vi "PeriodTasksNew.vi"() -> ()   [LabVIEW 2014]
panel:
  in  "Power Shaping Degree":dbl=2.0
  in  "Power Shaping Gain":dbl=50.0
  in  "Robot Width":dbl=27.25
  in  "Robot Length":dbl=19.875
  in  "Encoder Offset":dbl
  in  "EncoderTicksPerRev":dbl=1988.0
  in  "error in":errorcluster
  out "FL Angle":dbl=496.99998
  out "FR Angle":dbl=496.99998
  out "BL Angle":dbl=496.99998
  out "BR Angle":dbl=496.99998
  out "FL Power":dbl
  out "FR Power":dbl
  out "BL Power":dbl
  out "BR Power":dbl
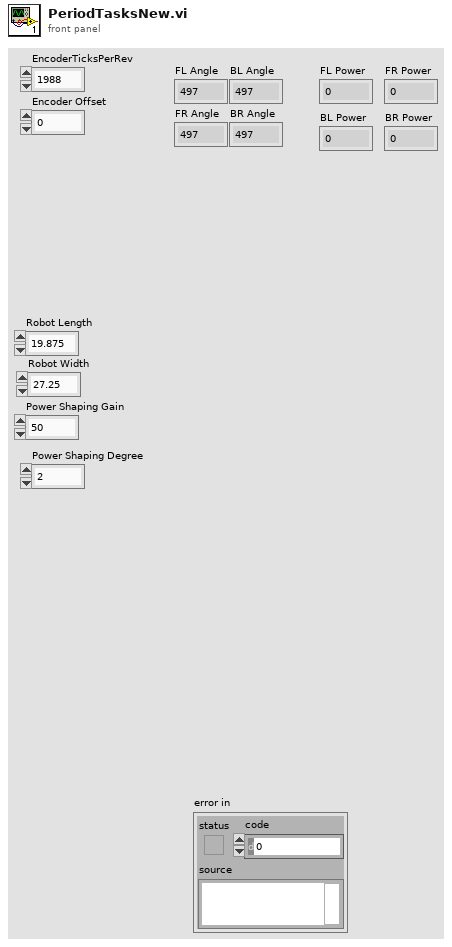
[diagram p1: front panel]
types:
  T1 = typedef "WPI_I2CDevRef.ctl" = cluster{"DevStatus":errorcluster, "Controller":T2, "Device Address":u8, "Handle":i32, "I2C Bus":T3}
  T2 = typedef "FPGA_TypedefDigitalModule.ctl" = enum16{"Controller 1"}
  T3 = typedef "i2c_bus.ctl" = enum16{"I2C On-Board", "I2C MXP", "Invalid"}
  T4 = typedef "WPI_MotorControlDeviceRef.ctl" = cluster{"DeviceStatus":errorcluster, "Type":T5, "PWM":cluster{"Controller":T2, "PWM Channel":T6, "DeadBand":T7}, "CAN":cluster{"Device Number":u8, "Control Mode":T8, "Semaphore":T9, "Max Vout":dbl, "TalonSRX Control Mode":T10}, "Invert":bool, "TransformRef":T11, "InvTransformRef":T11}
  T5 = typedef "WPI_MotorControlType.ctl" = enum16{"PWM", "CAN", "CANTalonSRX"}
  T6 = typedef "FPGA_DIOPWMChannel.ctl" = enum8{"PWM 0", "PWM 1", "PWM 2", "PWM 3", "PWM 4", "PWM 5", "PWM 6", "PWM 7", "PWM 8", "PWM 9", "PWM MXP 0", "PWM MXP 1", "PWM MXP 2", "PWM MXP 3", "PWM MXP 4", "PWM MXP 5", "PWM MXP 6", "PWM MXP 7", "PWM MXP 8", "PWM MXP 9", "Invalid"}
  T7 = typedef "WPI_PWMDeadband.ctl" = cluster{"Name":string, "maxPositivePwm":i32, "minPositivePwm":i32, "centerPwm":i32, "maxNegativePwm":i32, "minNegativePwm":i32, "angularRange":u16}
  T8 = typedef "WPI_CANJaguar_ControlMode.ctl" = enum8{"Percent VBus", "Current", "Speed", "Position", "Voltage"}
  T9 = typedef "Semaphore RefNum" = refnum<k1>
  T10 = typedef "WPI_CANTalonSRX_APIControlMode.ctl" = enum8{"Percent VBus", "Speed", "Position", "Slave", "Unchanged / Invalid"}
  T11 = typedef "WPI_PWMTransform_ConPane.ctl" = refnum<vi>
  T12 = typedef "WPI_JoystickDevRef.ctl" = cluster{"Device":T13}
  T13 = typedef "WPI_JoystickDeviceEnum.ctl" = enum16{"USB 0", "USB 1", "USB 2", "USB 3", "USB 4", "USB 5"}
  T14 = typedef "WPI_CANTalonSRX_GlobalStatus.ctl" = cluster{"Applied Throttle":dbl, "Module Enabled":bool, "CAN Error":errorcluster, "Closed Loop Error":dbl, "Forward Limit Switch Closed":bool, "Reverse Limit Switch Closed":bool, "Sensor Position":dbl, "Sensor Velocity":dbl, "Current":dbl, "Sticky Fault - Over Temp":bool, "Sticky Fault - Under Voltage":bool, "Sticky Fault - Forward Limit":bool, "Sticky Fault - Reverse Limit":bool, "Sticky Fault - Forward Soft Limit":bool, "Sticky Fault - Reverse Soft Limit":bool, "Brake is Enabled":bool, "Encoder Position":dbl, "Encoder Velocity":dbl, "Encoder Index Count":dbl, "Encoder A Pin State":bool, "Encoder B Pin State":bool, "Encoder Index Pin State":bool, "Analog In":dbl, "Analog In Velocity":dbl, "Temperature (C)":dbl, "Battery Voltage":dbl}
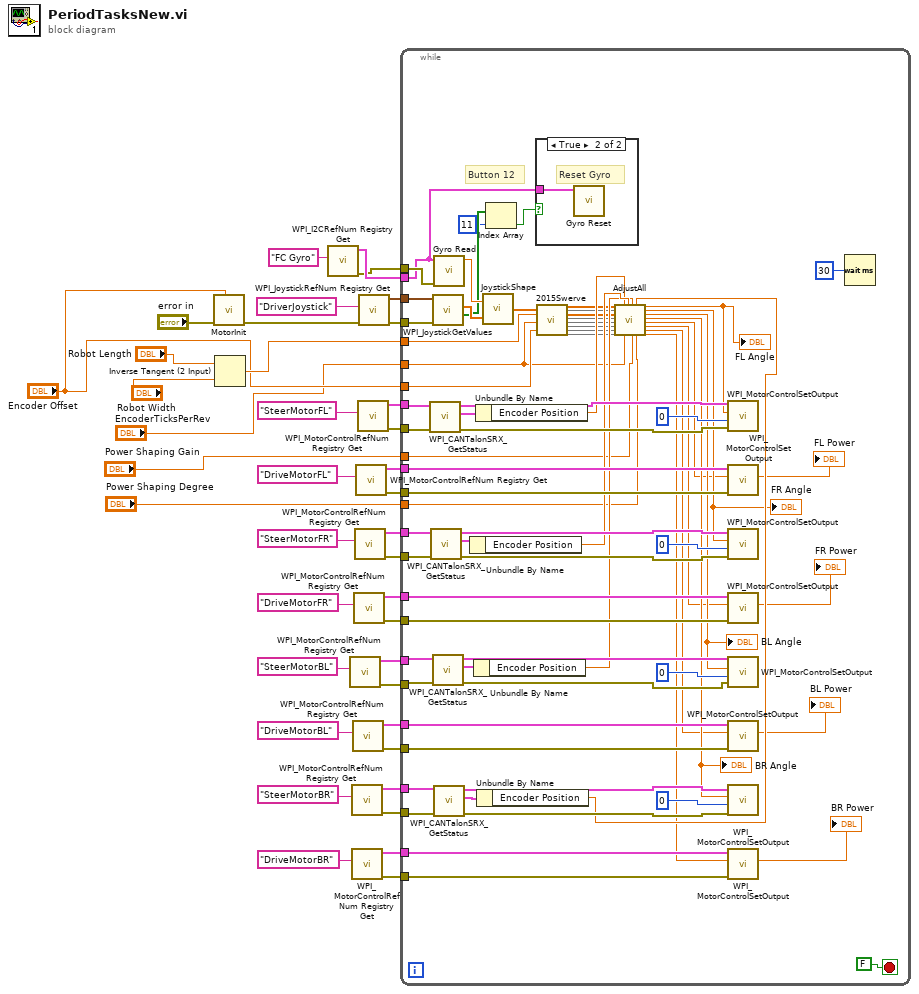
[diagram p0: block diagram]
diagram:
  n1 = call "MotorInit.vi"("Encoder Initial Position"="Encoder Offset", "error in"="error in") -> ("error out"=w10:errorcluster)  [unwired: 9 in]
  n2 = Inverse Tangent (2 Input)(1:"Robot Width", 2:"Robot Length") -> (0:w12:dbl)
  n3 = call <vilib>:"WPI_I2CRefNum Registry Get.vi"("refnum name"="FC Gyro") -> ("error out"=w1:errorcluster, "I2CDevRef"=w6:T1)  [unwired: 9 in]
  n4 = call <vilib>:"WPI_MotorControlRefNum Registry Get.vi"("refnum name"="SteerMotorBL") -> ("error out"=w20:errorcluster, "MotorControlDevRef"=w21:T4)  [unwired: 9 in]
  n5 = call <vilib>:"WPI_MotorControlRefNum Registry Get.vi"("refnum name"="SteerMotorBR") -> ("error out"=w15:errorcluster, "MotorControlDevRef"=w16:T4)  [unwired: 9 in]
  n6 = call <vilib>:"WPI_MotorControlRefNum Registry Get.vi"("refnum name"="DriveMotorBR") -> ("error out"=w13:errorcluster, "MotorControlDevRef"=w14:T4)  [unwired: 9 in]
  n7 = call <vilib>:"WPI_MotorControlRefNum Registry Get.vi"("refnum name"="DriveMotorBL") -> ("error out"=w17:errorcluster, "MotorControlDevRef"=w18:T4)  [unwired: 9 in]
  n8 = call <vilib>:"WPI_MotorControlRefNum Registry Get.vi"("refnum name"="DriveMotorFR") -> ("error out"=w22:errorcluster, "MotorControlDevRef"=w23:T4)  [unwired: 9 in]
  n9 = call <vilib>:"WPI_MotorControlRefNum Registry Get.vi"("refnum name"="SteerMotorFR") -> ("error out"=w24:errorcluster, "MotorControlDevRef"=w25:T4)  [unwired: 9 in]
  n10 = call <vilib>:"WPI_MotorControlRefNum Registry Get.vi"("refnum name"="DriveMotorFL") -> ("error out"=w26:errorcluster, "MotorControlDevRef"=w27:T4)  [unwired: 9 in]
  n11 = call <vilib>:"WPI_MotorControlRefNum Registry Get.vi"("refnum name"="SteerMotorFL") -> ("error out"=w28:errorcluster, "MotorControlDevRef"=w29:T4)  [unwired: 9 in]
  n12 = call <vilib>:"WPI_JoystickRefNum Registry Get.vi"("error in (no error)"=w10, "refnum name"="DriverJoystick") -> ("error out"=w11:errorcluster, "JoystickDevRef"=w37:T12)  [unwired: 8 in]
  n13 = while {
    tunnel: w37 -> [w107]
    tunnel: w11 -> [w106]
    tunnel: w29 -> [w89]
    tunnel: w28 -> [w87]
    tunnel: w27 -> [w100]
    tunnel: w26 -> [w99]
    tunnel: w25 -> [w84]
    tunnel: w24 -> [w83]
    tunnel: w23 -> [w97]
    tunnel: w22 -> [w96]
    tunnel: w21 -> [w79]
    tunnel: w20 -> [w78]
    tunnel: w18 -> [w94]
    tunnel: w17 -> [w93]
    tunnel: w16 -> [w74]
    tunnel: w15 -> [w73]
    tunnel: w14 -> [w91]
    tunnel: w13 -> [w90]
    tunnel: w12 -> [w103]
    tunnel: "EncoderTicksPerRev" -> [w47]
    tunnel: "Encoder Offset" -> [w49]
    tunnel: w6 -> [w43]
    tunnel: "Power Shaping Gain" -> [w46]
    tunnel: "Power Shaping Degree" -> [w45]
    tunnel: w1 -> [w44]
    stop <- FALSE stop-if-true
    # "Button 12"
    n14 = call <vilib>:"WPI_CANTalonSRX_GetStatus.vi"("error in (no error)"=w87, "CAN Talon SRX Ref"=w89) -> ("error out"=w86:errorcluster, "Talon SRX Status"=w85:T14, "CAN Talon SRX Ref Out"=w88:T4)  [unwired: 7 in]
    n15 = call <vilib>:"WPI_CANTalonSRX_GetStatus.vi"("error in (no error)"=w83, "CAN Talon SRX Ref"=w84) -> ("error out"=w81:errorcluster, "Talon SRX Status"=w80:T14, "CAN Talon SRX Ref Out"=w82:T4)  [unwired: 7 in]
    n16 = call <vilib>:"WPI_JoystickGetValues.vi"("error in (no error)"=w106, "JoystickDevRef"=w107) -> ("Buttons"=w41:bool[], "Axes"=w105:dbl[])  [unwired: 5 in, 3 out]
    n17 = call <vilib>:"WPI_CANTalonSRX_GetStatus.vi"("error in (no error)"=w78, "CAN Talon SRX Ref"=w79) -> ("error out"=w76:errorcluster, "Talon SRX Status"=w75:T14, "CAN Talon SRX Ref Out"=w77:T4)  [unwired: 7 in]
    n18 = call "Gyro Read.vi"("error in (no error)"=w44, "I2CDevRef In"=w43) -> ("Angle"=w48:dbl)  [unwired: 7 in, 2 out]
    n19 = call <vilib>:"WPI_CANTalonSRX_GetStatus.vi"("error in (no error)"=w73, "CAN Talon SRX Ref"=w74) -> ("error out"=w71:errorcluster, "Talon SRX Status"=w70:T14, "CAN Talon SRX Ref Out"=w72:T4)  [unwired: 7 in]
    n20 = Unbundle By Name(w80) -> ("Encoder Position"=w69:dbl)
    n21 = Unbundle By Name(w75) -> ("Encoder Position"=w67:dbl)
    n22 = Unbundle By Name(w85) -> ("Encoder Position"=w68:dbl)
    n23 = Unbundle By Name(w70) -> ("Encoder Position"=w66:dbl)
    n24 = call "JoystickShape.vi"("JoystickValues"=w105, "Gyro"=w48) -> ("JoystickOut"=w104:dbl[])
    n25 = Index Array(array=w41, index=11) -> (element=w42:bool)
    n26 = case shown="True" w42 {
      tunnel: w43 -> [_ w109]
      frame False {
      }
      frame True {
        # "Reset Gyro"
        n27 = call "Gyro Reset.vi"("I2CDevRef"=w109) -> ()  [unwired: 10 in, 1 out]
      }
    }
    n28 = call "2015Swerve.vi"("Axes"=w104, "Robot Dimension Calc"=w103, "EncoderTicksPerRev"=w47, "Encoder Offset"=w49) -> ("SteeringArray"=w65:dbl[], 21:w64, "PowerArray"=w63:dbl[], 23:w62, 24:w61, 25:w60, 26:w59, 27:w58)  [unwired: 16 in]
    n29 = call "AdjustAll.vi"("SteeringAngleArray"=w65, 1:w64, "PowerArray"=w63, 3:w62, 4:w61, 5:w60, 6:w59, 7:w58, "FL Enc"=w68, "EncoderTicksPerRev"=w47, "FR Enc"=w69, "BL Enc"=w67, "Gain"=w46, "BR Enc"=w66, "Shaping Degree"=w45) -> ("FL Set Out"=w57:dbl, "FR Set Out"=w56:dbl, "BL Set Out"=w55:dbl, "BR Set Out"=w54:dbl, "FL Power"=w53:dbl, "FR Power"=w52:dbl, "BL Power"=w51:dbl, "BR Power"=w50:dbl)  [unwired: 5 in]
    "FL Angle" <- w57
    "FR Angle" <- w56
    "BL Angle" <- w55
    "BR Angle" <- w54
    "FL Power" <- w53
    "FR Power" <- w52
    "BL Power" <- w51
    "BR Power" <- w50
    n30 = call <vilib>:"WPI_MotorControlSetOutput.vi"("error in (no error)"=w86, "Sync Group / Parameter Slot"=u8 0, "Output"=w57, "MotorControlDevRef"=w88) -> ()  [unwired: 5 in, 3 out]
    n31 = call <vilib>:"WPI_MotorControlSetOutput.vi"("error in (no error)"=w99, "Output"=w53, "MotorControlDevRef"=w100) -> ()  [unwired: 6 in, 3 out]
    n32 = call <vilib>:"WPI_MotorControlSetOutput.vi"("error in (no error)"=w81, "Sync Group / Parameter Slot"=u8 0, "Output"=w56, "MotorControlDevRef"=w82) -> ()  [unwired: 5 in, 3 out]
    n33 = call <vilib>:"WPI_MotorControlSetOutput.vi"("error in (no error)"=w96, "Output"=w52, "MotorControlDevRef"=w97) -> ()  [unwired: 6 in, 3 out]
    n34 = call <vilib>:"WPI_MotorControlSetOutput.vi"("error in (no error)"=w76, "Sync Group / Parameter Slot"=u8 0, "Output"=w55, "MotorControlDevRef"=w77) -> ()  [unwired: 5 in, 3 out]
    n35 = call <vilib>:"WPI_MotorControlSetOutput.vi"("error in (no error)"=w93, "Output"=w51, "MotorControlDevRef"=w94) -> ()  [unwired: 6 in, 3 out]
    n36 = call <vilib>:"WPI_MotorControlSetOutput.vi"("error in (no error)"=w71, "Sync Group / Parameter Slot"=u8 0, "Output"=w54, "MotorControlDevRef"=w72) -> ()  [unwired: 5 in, 3 out]
    n37 = call <vilib>:"WPI_MotorControlSetOutput.vi"("error in (no error)"=w90, "Output"=w50, "MotorControlDevRef"=w91) -> ()  [unwired: 6 in, 3 out]
    n38 = Wait (ms)(milliseconds to wait=u32 30) -> ()  [unwired: 1 out]
  }
